vi "ReadStatusByte.vi"(2 "unsigned byte array":u8[](array[numeric])) -> (5 "Specifier Status":bool, 6 "Command not accepted":bool, 7 "Units":string="um", 8 "Action required":bool, 9 "Direction":string="um", 10 "Scan direction":string="um")   [LabVIEW 2017, in "Spectral Products CM110.lvlib"]
uses:
  Spectral Products CM110.lvlib
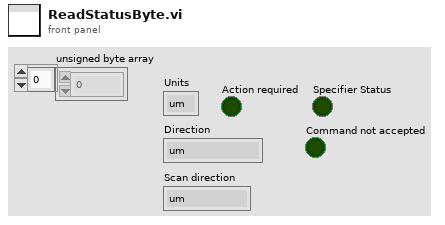
[diagram p1: front panel]
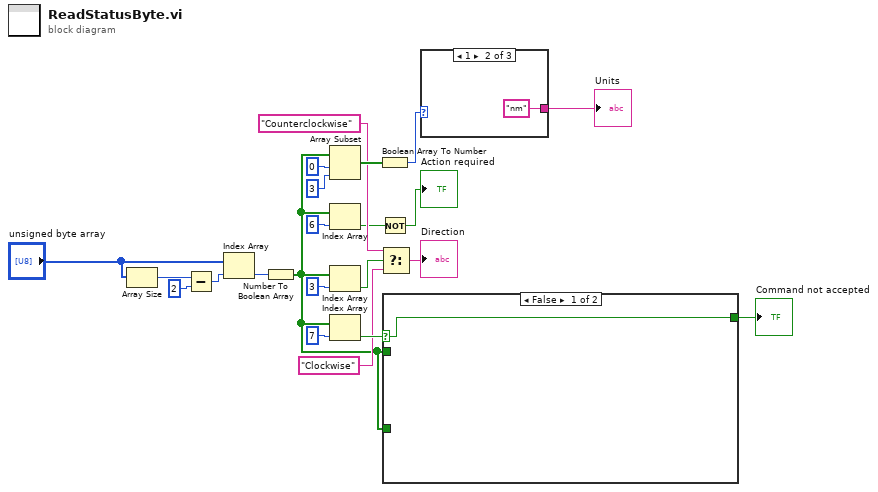
[diagram p0: block diagram]
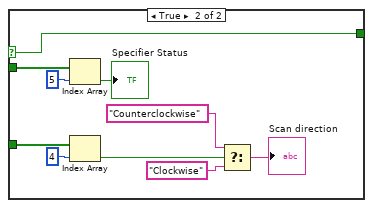
[diagram p2: hidden frame]
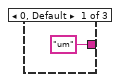
[diagram p3: hidden frame]
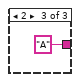
[diagram p4: hidden frame]
diagram:
  n1 = Array Size(array="unsigned byte array") -> (size(s)=w20:i32)
  n2 = Subtract(x=w20, y=2) -> (x-y=w22:i32)
  n3 = Index Array(array="unsigned byte array", index=w22) -> (element=w19:u8)
  n4 = Number To Boolean Array(number=w19) -> (Boolean array=w4:bool[])
  n5 = Array Subset(array=w4, index=0, length=3) -> (w15:bool[])
  n6 = Index Array(array=w4, index=6) -> (element=w3:bool)
  n7 = Index Array(array=w4, index=3) -> (element=w11:bool)
  n8 = Index Array(array=w4, index=7) -> (element=w7:bool)
  n9 = Boolean Array To Number(Boolean array=w15) -> (number=w14:u32)
  n10 = Not(x=w3) -> (.not. x?=→"Action required":bool)
  n11 = Select(t="Counterclockwise", s=w11, f="Clockwise") -> (s? t:f=→"Direction":string)
  n12 = case shown="False" w7 {
    selector: w7 -> [w23 w24]
    tunnel: w4 -> [_ w33]
    tunnel: w4 -> [_ w26]
    tunnel: [w23 w24] -> w1
    frame False {
    }
    frame True {
      n13 = Index Array(array=w26, index=5) -> (element=→"Specifier Status":bool)
      n14 = Index Array(array=w33, index=4) -> (element=w28:bool)
      n15 = Select(t="Counterclockwise", s=w28, f="Clockwise") -> (s? t:f=→"Scan direction":string)
    }
  }
  "Command not accepted" <- w1
  n16 = case shown="1" w14 {
    tunnel: ["um" "nm" "A"] -> w13
    frame 0, Default {
    }
    frame 1 {
    }
    frame 2 {
    }
  }
  "Units" <- w13
